vi "Read buffer.vi"(8 "error in (no error)":errorcluster, 11 "httpRequest in":refnum<class "httpRequest.lvclass">) -> (0 "error out":errorcluster, 2 "buffer":string, 3 "httpRequest out":refnum<class "httpRequest.lvclass">)   [LabVIEW 2020, in "httpClient.lvlib" / "httpRequest.lvclass"]
uses:
  httpRequest.lvclass
  httpRequest.lvclass/httpRequest.ctl
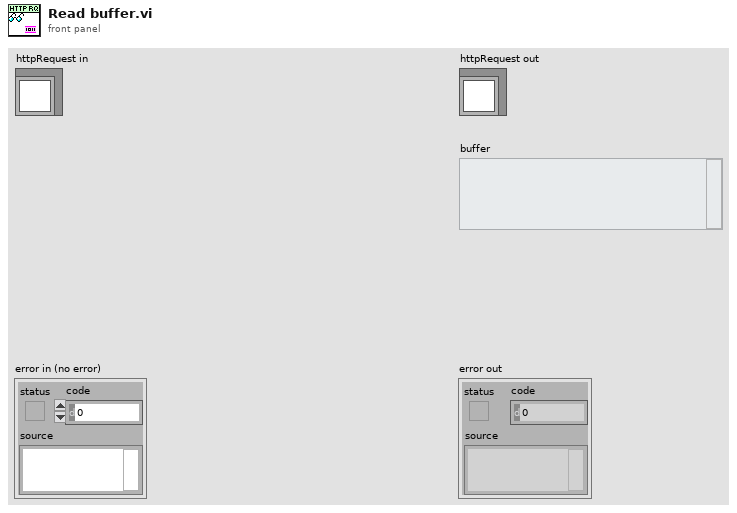
[diagram p1: front panel]
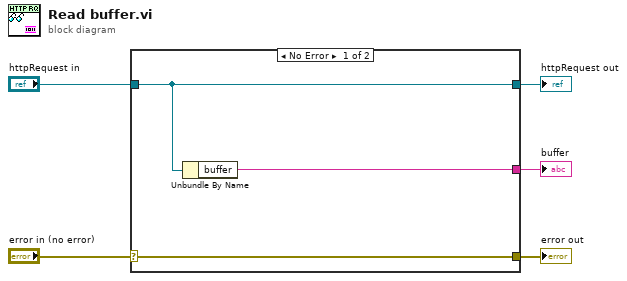
[diagram p0: block diagram]
diagram:
  n1 = case shown="No Error" "error in (no error)" {
    selector: "error in (no error)" -> [w8 w9]
    tunnel: [w8 w9] -> w4
    tunnel: [w7 w10] -> w2
    tunnel: "httpRequest in" -> [w7 w10]
    tunnel: [w6 _] -> w1
    frame No Error {
      n2 = Unbundle By Name(w7) -> ("buffer"=w6:string)
    }
    frame Error {
    }
  }
  "error out" <- w4
  "httpRequest out" <- w2
  "buffer" <- w1
